vi "poly_fit.vi"(9 "liczba probek":dbl, 10 "PIEZO":dbl[](array[numeric])) -> (2 "fitted piezo":dbl[](array[numeric]))   [LabVIEW 2013]
uses:
  <vilib>/Analysis/6fits.llb/Curve Fitting Criteria.ctl
  <vilib>/Analysis/1siggen.llb/Ramp Pattern by Samples.vi
  <vilib>/Analysis/NI_AALBase.lvlib
  <vilib>/Analysis/NI_AALPro.lvlib
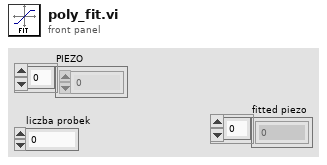
[diagram p1: front panel]
types:
  T1 = typedef "NI_AALPro.lvlib/Curve Fitting Criteria.ctl" = u16
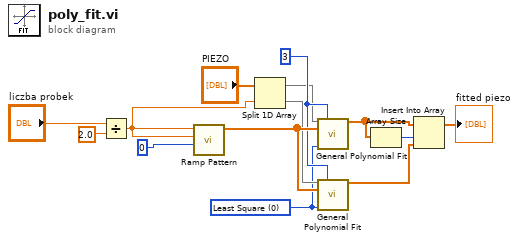
[diagram p0: block diagram]
diagram:
  w1 = T1 0 items=["Least Square", "Least Absolute Residual", "Bisquare"] ("method")
  w9 = 3
  n1 = Divide(x="liczba probek", y=2.0) -> (x/y=w12:dbl)
  n2 = call-poly <vilib>:"Ramp Pattern.vi"("start"=0, "end"=w12, "samples"=w12) -> ("Ramp Pattern"=w13:dbl[])  [unwired: 7 in, 1 out]
  n3 = Split 1D Array(array="PIEZO", index=w12) -> (first subarray=w6:dbl[], second subarray=w8:dbl[])
  n4 = call <vilib>:"General Polynomial Fit.vi"("Y"=w6, "polynomial order"=w9, "X"=w13, "method"=w1) -> ("Best Polynomial Fit"=w3:dbl[])  [unwired: 8 in, 3 out]
  n5 = call <vilib>:"General Polynomial Fit.vi"("Y"=w8, "polynomial order"=w9, "X"=w13, "method"=w1) -> ("Best Polynomial Fit"=w2:dbl[])  [unwired: 8 in, 3 out]
  n6 = Array Size(array=w3) -> (size(s)=w5:i32)
  n7 = Insert Into Array(array=w3, index=w5, new element=w2) -> (→"fitted piezo":dbl[])
